vi "Get.vi"() -> ()   [LabVIEW 2020]
uses:
  <vilib>/httpClient/LabVIEWHTTPClient.lvlib
panel:
  out "error out":errorcluster
  out "body":string
  out "headers":string
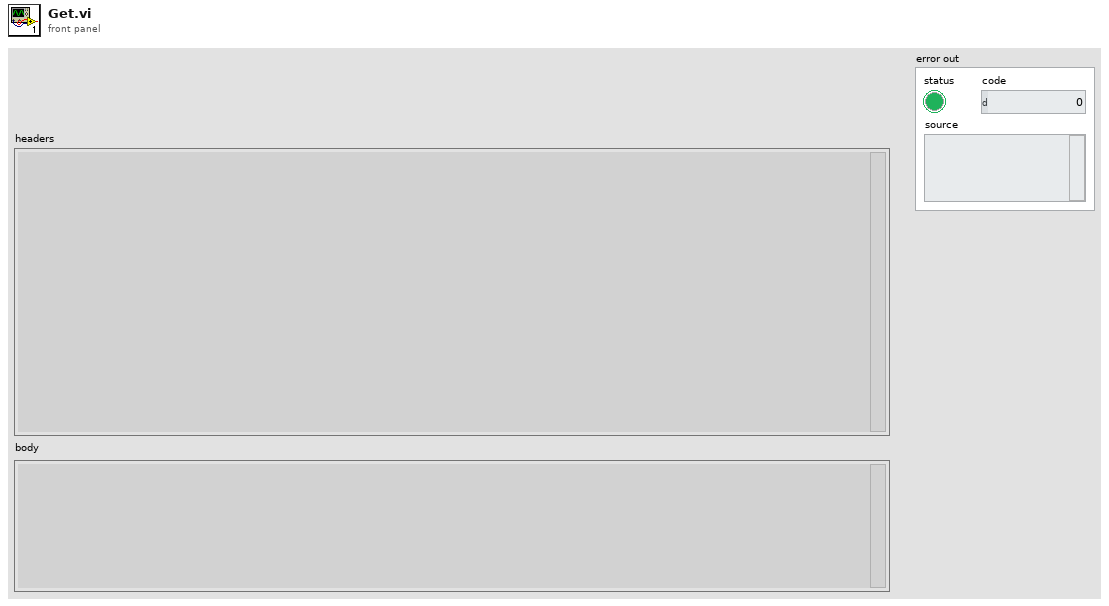
[diagram p1: front panel]
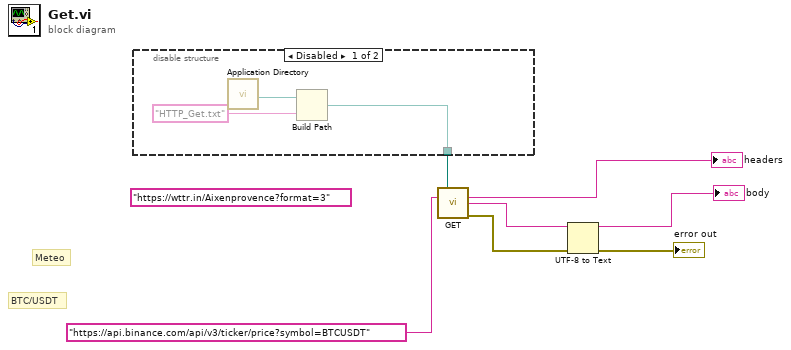
[diagram p0: block diagram]
diagram:
  (unwired) "https://wttr.in/Aixenprovence?format=3" ("url")
  # "BTC/USDT"
  # "Meteo"
  n1 = disable-structure shown="Disabled" {
    disable-tunnel: [w10 _] -> w6
    frame Disabled {
      n2 = call <vilib>:"Application Directory.vi"() -> ("Application Directory"=w9:path)
      n3 = Build Path(base path=w9, name or relative path="HTTP_Get.txt") -> (appended path=w10:path)
    }
    frame Enabled {
    }
  }
  n4 = call <vilib>:"GET.vi"("output file"=w6, "url"="https://api.binance.com/api/v3/ticker/price?symbol=BTCUSDT") -> ("headers"=→"headers":string, "body"=w3:string, "error out"=w5:errorcluster)  [unwired: 10 in, 1 out]
  n5 = UTF-8 to Text(8:w5, 11:w3) -> (0:→"error out":errorcluster, 3:→"body":string)  [unwired: 1 in]
